vi "Make New Set.vi"() -> ()   [LabVIEW 2010, in "TemplateGenerator.lvlib"]
uses:
  TemplateGenerator.lvlib
panel:
  in  "Library Path":path=path "C:/perforce/Sales/projects/Components/Current Value Table (CVT)/3.x/CVT3/Current Value Table.lvlib"
  in  "Control Path":path
  in  "Color":u32(colorbox)
  in  "3-Char Type":string
  in  "Data Type":string
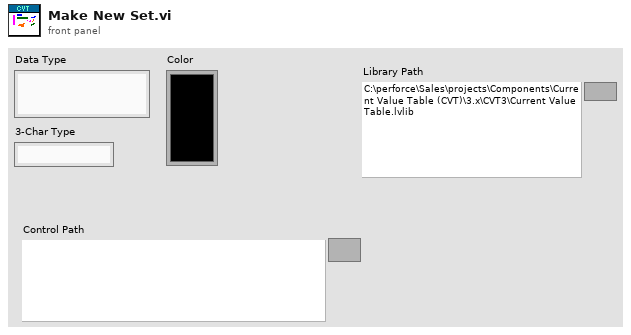
[diagram p1: front panel]
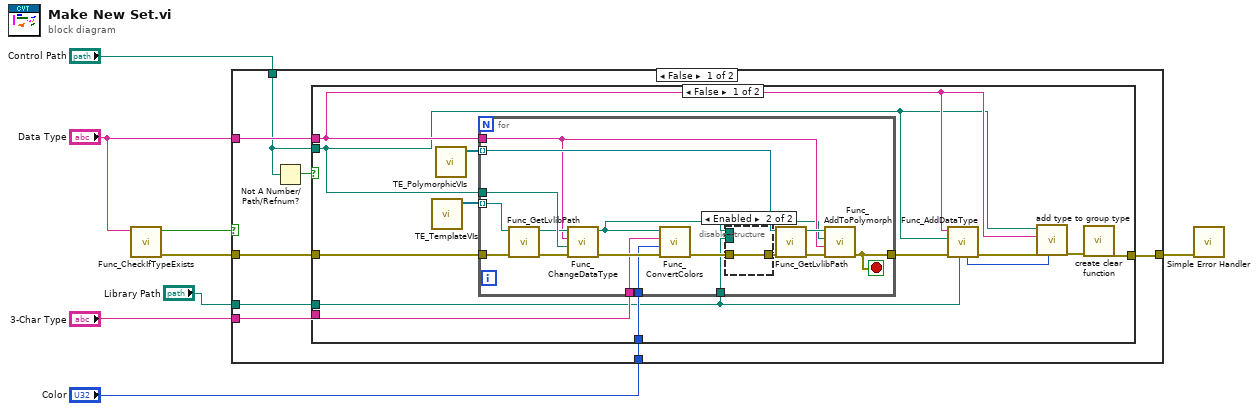
[diagram p0: block diagram]
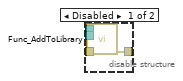
[diagram p2: hidden frame]
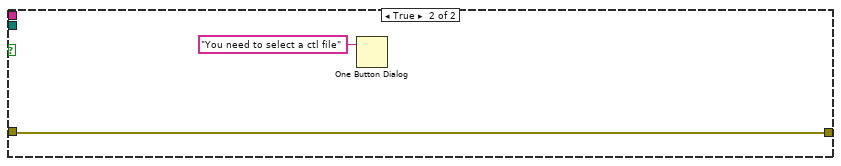
[diagram p3: hidden frame]
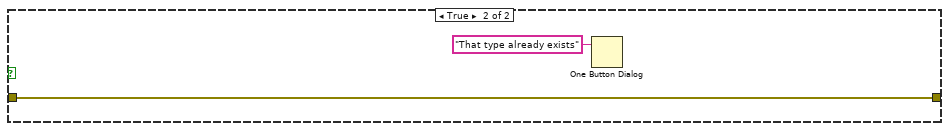
[diagram p4: hidden frame]
diagram:
  n1 = call "Func_CheckIfTypeExists.vi"("data type name"="Data Type") -> ("error out"=w7:errorcluster, "Exists"=w3:bool)  [unwired: 9 in]
  n2 = case shown="False" w3 {
    tunnel: [w15 w54] -> w8
    tunnel: "Data Type" -> [w14 _]
    tunnel: w7 -> [w16 w54]
    tunnel: "Color" -> [w13 _]
    tunnel: "3-Char Type" -> [w12 _]
    tunnel: "Control Path" -> [w11 _]
    tunnel: "Library Path" -> [w9 _]
    frame False {
      n3 = Not A Number/Path/Refnum?(number/path/refnum=w11) -> (NaN/Path/Refnum?=w10:bool)
      n4 = case shown="False" w10 {
        tunnel: w16 -> [w27 w53]
        tunnel: w11 -> [w21 _]
        tunnel: [w19 w53] -> w15
        tunnel: w14 -> [w22 _]
        tunnel: w13 -> [w25 _]
        tunnel: w12 -> [w24 _]
        tunnel: w9 -> [w17 _]
        frame False {
          n5 = call "TE_TemplateVIs.vi"() -> ("VI References"=w29:refnum<vi>[])  [unwired: 11 in]
          n6 = call "TE_PolymorphicVIs.vi"() -> ("VI References"=w28:refnum<vi>[])  [unwired: 11 in]
          n7 = for {
            tunnel: w21 -> [w46]
            tunnel: w27 -> [w43]
            tunnel: w22 -> [w36]
            tunnel: w29 -> [w44] mode=indexing
            tunnel: w28 -> [w39] mode=indexing
            tunnel: [w45] -> w26
            tunnel: w25 -> [w32]
            tunnel: w24 -> [w31]
            tunnel: w17 -> [w30]
            stop <- w45 stop-if-true
            n8 = call "Func_GetLvlibPath.vi"("error in (no error)"=w43, "VI in"=w44) -> ("error out"=w41:errorcluster, "VI Path"=w42:path)  [unwired: 8 in]
            n9 = call "Func_ChangeDataType.vi"("error in (no error)"=w41, "Control Path"=w46, "data type name"=w36, "template"=w42) -> ("error out"=w34:errorcluster, "Final Path"=w35:path)  [unwired: 6 in]
            n10 = call "Func_ConvertColors.vi"("error in (no error)"=w34, "Color Box"=w32, "New Type"=w31, "Path"=w35) -> ("error out"=w33:errorcluster)  [unwired: 7 in]
            n11 = disable-structure shown="Enabled" {
              disable-tunnel: [w50 w51] -> w40
              disable-tunnel: w35 -> [w49 _]
              disable-tunnel: w33 -> [w48 w51]
              disable-tunnel: w30 -> [w47 _]
              frame Disabled {
                n12 = call "Func_AddToLibrary.vi"("error in (no error)"=w48, "Library Path"=w47, "VI Path"=w49) -> ("error out"=w50:errorcluster)  [unwired: 8 in]
              }
              frame Enabled {
              }
            }
            n13 = call "Func_GetLvlibPath.vi"("error in (no error)"=w40, "VI in"=w39) -> ("error out"=w37:errorcluster, "VI Path"=w38:path)  [unwired: 8 in]
            n14 = call "Func_AddToPolymorph.vi"("error in (no error)"=w37, "Name"=w36, "New VI's Path"=w35, "Polymorphic VI Path"=w38) -> ("error out"=w45:errorcluster)  [unwired: 6 in, 1 out]
          }
          n15 = call "Func_AddDataType.vi"("Library Path"=w17, "error in (no error)"=w26, "Control Path"=w21, "data type name"=w22) -> ("error out"=w23:errorcluster, "Polymorph count"=w20:i32)  [unwired: 6 in]
          n16 = call "add type to group type.vi"("Selected Type"=w20, "error in (no error)"=w23, "Data Type"=w22, "Control Path"=w21) -> ("error out"=w18:errorcluster)  [unwired: 7 in]
          n17 = call "create clear function.vi"("error in (no error)"=w18) -> ("error out"=w19:errorcluster)  [unwired: 10 in]
        }
        frame True {
          n18 = One Button Dialog(message="You need to select a ctl file") -> ()  [unwired: 1 in, 1 out]
        }
      }
    }
    frame True {
      n19 = One Button Dialog(message="That type already exists") -> ()  [unwired: 1 in, 1 out]
    }
  }
  n20 = call <vilib>:"Simple Error Handler.vi"("error in (no error)"=w8) -> ()  [unwired: 4 in, 5 out]
